vi "createDataFolder.vi"() -> ()   [LabVIEW 2018]
panel:
  out "创建的路径 CH2":path
  out "创建的路径 CH1":path
  out "CH2索引":i32
  out "CH1索引":i32
  out "文件夹名":string[](array[string])
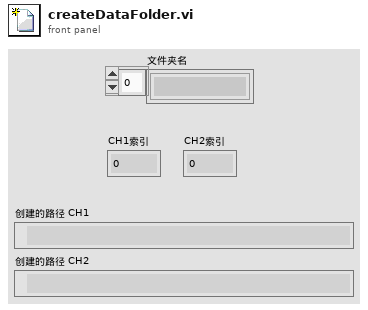
[diagram p1: front panel]
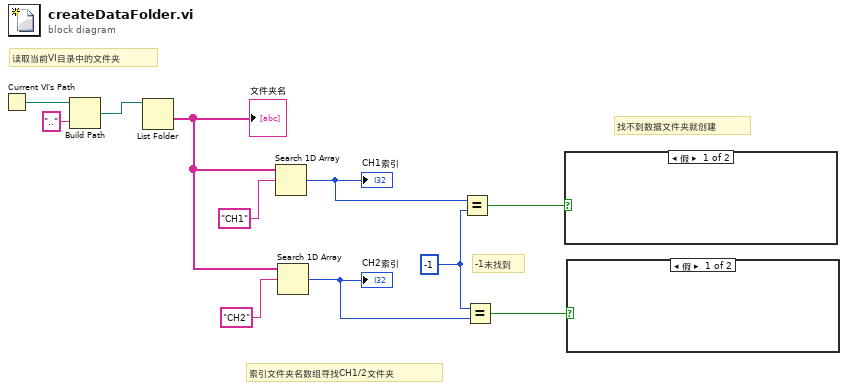
[diagram p0: block diagram]
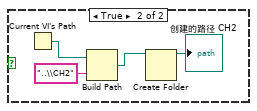
[diagram p2: hidden frame]
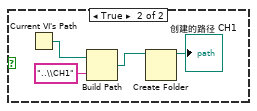
[diagram p3: hidden frame]
diagram:
  w4 = -1 ("x")
  # "找不到数据文件夹就创建"
  # "-1未找到"
  # "索引文件夹名数组寻找CH1/2文件夹"
  # "读取当前VI目录中的文件夹"
  n1 = Current VI's Path() -> (path=w11:path)
  n2 = Build Path(base path=w11, name or relative path=".." ("名称或相对路径")) -> (appended path=w2:path)
  n3 = List Folder(path=w2) -> (folder names=w7:string[])  [unwired: 3 in, 3 out]
  "文件夹名" <- w7
  n4 = Search 1D Array(1D array=w7, element="CH1" ("元素")) -> (index of element=w6:i32)  [unwired: 1 in]
  "CH1索引" <- w6
  n5 = Search 1D Array(1D array=w7, element="CH2" ("元素")) -> (index of element=w5:i32)  [unwired: 1 in]
  "CH2索引" <- w5
  n6 = Equal?(x=w6, y=w4) -> (x = y?=w3:bool)
  n7 = Equal?(x=w4, y=w5) -> (x = y?=w1:bool)
  n8 = case shown="假" w3 {
    frame False {
    }
    frame True {
      n9 = Current VI's Path() -> (path=w12:path)
      n10 = Build Path(base path=w12, name or relative path="..\\CH1" ("名称或相对路径")) -> (appended path=w14:path)
      n11 = Create Folder(path (use dialog)=w14) -> (created path=→"创建的路径 CH1":path)  [unwired: 2 in, 2 out]
    }
  }
  n12 = case shown="假" w1 {
    frame False {
    }
    frame True {
      n13 = Current VI's Path() -> (path=w16:path)
      n14 = Build Path(base path=w16, name or relative path="..\\CH2" ("名称或相对路径")) -> (appended path=w18:path)
      n15 = Create Folder(path (use dialog)=w18) -> (created path=→"创建的路径 CH2":path)  [unwired: 2 in, 2 out]
    }
  }
